vi "RPTID Manager.vi"(8 "error in (no error)":errorcluster, 11 "RPTID Data":cluster{"RPTID":u32, "VID":u32[]}[](array[cluster])) -> (0 "error out":errorcluster)   [LabVIEW 2020, in "SECS Scenarios.lvlib" / "33-RPTID Setup.lvclass"]
uses:
  33-RPTID Setup.lvclass
  SECS Communication/SECS Data Class/RPTID Data.ctl
  SECS Communication/SECS Data Class/Remove RPTID.vi
  SECS Communication/SECS Data Class/Add RPTID.vi
  SECS Communication/SECS Data Class/Get All RPTID Data.vi
  SECS Communication/SECS Data Class/SECS Data Class.lvclass
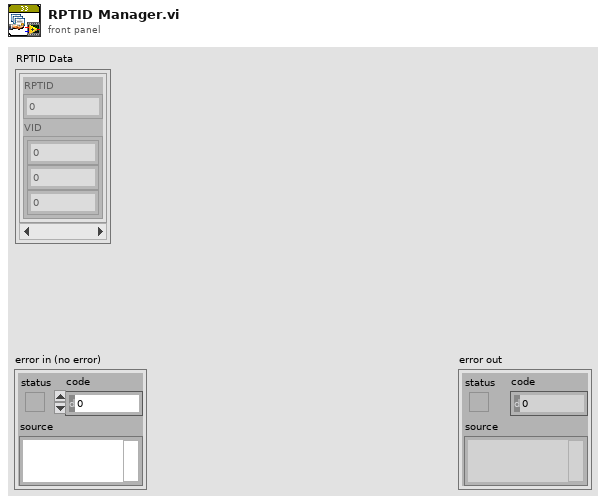
[diagram p1: front panel]
types:
  T1 = typedef "SECS Communication.lvlib/SECS Data Class.lvclass/RPTID Data.ctl" = cluster{"RPTID":u32, "Report Information":string[], "Dynamic":bool}
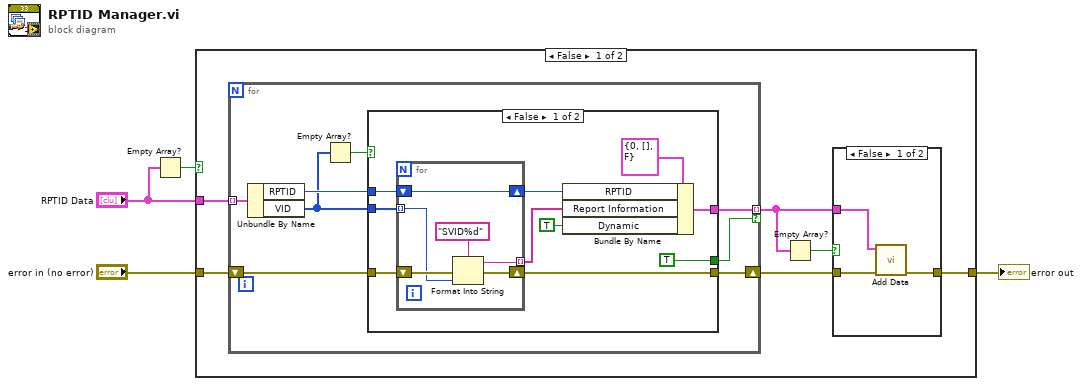
[diagram p0: block diagram]
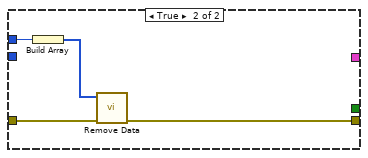
[diagram p3: hidden frame]
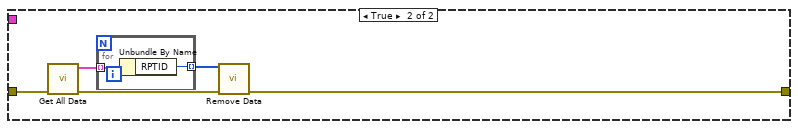
[diagram p4: hidden frame]
diagram:
  n1 = Empty Array?(array="RPTID Data") -> (empty?=w1:bool)
  n2 = case shown="False" w1 {
    tunnel: "error in (no error)" -> [w10 w47]
    tunnel: [w7 w43] -> w3
    tunnel: "RPTID Data" -> [w9 _]
    frame False {
      n3 = for {
        tunnel: w9 -> [w22] mode=indexing
        shift-right: [w19] -> w8
        shift-left: w10 -> [w20]
        tunnel: [w18] -> w6 mode=indexing if=w15
        n4 = Unbundle By Name(w22) -> ("RPTID"=w21:u32, "VID"=w17:u32[])
        n5 = Empty Array?(array=w17) -> (empty?=w16:bool)
        n6 = case shown="False" w16 {
          tunnel: w21 -> [w32 w42]
          tunnel: w20 -> [w31 w41]
          tunnel: [w27 w39] -> w19
          tunnel: [w26 _] -> w18
          tunnel: w17 -> [w25 _]
          tunnel: [TRUE _] -> w15
          frame False {
            n7 = for {
              shift-right: [w33] -> w29
              shift-left: w32 -> [w33]
              tunnel: w25 -> [w37] mode=indexing
              tunnel: [w34] -> w28 mode=indexing
              shift-right: [w35] -> w27
              shift-left: w31 -> [w38]
              n8 = Format Into String(format string="SVID%d", error in=w38, w37) -> (resulting string=w34:string, error out=w35:errorcluster)  [unwired: 1 in]
            }
            n9 = Bundle By Name(cluster=T1 {"RPTID"=0, "Report Information"=[], "Dynamic"=FALSE} ("RPTID Data"), "RPTID"=w29, "Report Information"=w28, "Dynamic"=TRUE) -> (w26:T1)
          }
          frame True {
            n10 = Build Array(w42) -> (w40:u32[])
            n11 = call-poly "Remove Data.vi"("error in (no error)"=w41, "RPTID"=w40) -> ("error out"=w39:errorcluster)  [unwired: 9 in]
          }
        }
      }
      n12 = Empty Array?(array=w6) -> (empty?=w5:bool)
      n13 = case shown="False" w5 {
        tunnel: w8 -> [w13 w14]
        tunnel: [w12 w14] -> w7
        tunnel: w6 -> [w11 _]
        frame False {
          n14 = call-poly "Add Data.vi"("error in (no error)"=w13, "RPTID Data In"=w11) -> ("error out"=w12:errorcluster)  [unwired: 9 in]
        }
        frame True {
        }
      }
    }
    frame True {
      n15 = call-poly "Get All Data.vi"("error in (no error)"=w47) -> ("error out"=w45:errorcluster, "RPTID Data"=w46:T1[])  [unwired: 9 in]
      n16 = for {
        tunnel: w46 -> [w49] mode=indexing
        tunnel: [w48] -> w44 mode=indexing
        n17 = Unbundle By Name(w49) -> ("RPTID"=w48:u32)
      }
      n18 = call-poly "Remove Data.vi"("error in (no error)"=w45, "RPTID"=w44) -> ("error out"=w43:errorcluster)  [unwired: 9 in]
    }
  }
  "error out" <- w3
